vi "LSMcontroller_v63_3Dfocus.vi"() -> ()   [LabVIEW 2015] (continued)
                    n3072 = property on="save\ndata" class="Bool (strict)"("DisabledEnum"=T7."Enabled" ("Disabled")) -> ()  [unwired: 2 in, 2 out]
                    n3073 = property on="save\ndata" class="Bool (strict)"("Value"=TRUE ("save\ndata")) -> ()  [unwired: 2 in, 2 out]
                    n3074 = property on="# of frames" class="DigNum (strict)"("DisabledEnum"=T7."Enabled" ("Disabled")) -> ()  [unwired: 2 in, 2 out]
                  }
                }
              }
              frame #1 {
                n3075 = local read "finite samples"() -> (w6248:bool)
                n3076 = local read "continuous"() -> (w6247:bool)
                n3077 = local read "wavdet"() -> (w6246:bool)
                n3078 = call "2pparameters.vi"("command"="get") -> ("params out"=w6242:T10)  [unwired: 1 in]
                n3079 = Bundle By Name(cluster=w6242, "finite"=w6248, "cont"=w6247, "wavdet"=w6246) -> (w6245:T10)
                n3080 = call "2pparameters.vi"("Params in"=w6245, "command"="set") -> ()  [unwired: 1 out]
              }
            }
          }
          event "continuous": Value Change {
            n3081 = event-data() -> ("NewVal"=w6249:bool)  [unwired: 1 in]
            n3082 = flat-sequence {
              tunnel: w6249 -> [w6250]
              frame #0 {
                n3083 = case shown="True" w6250 {
                  frame False {
                    n3084 = property on="finite samples" class="Bool (strict)"("Value"=TRUE ("finite samples for recording")) -> ()  [unwired: 2 in, 2 out]
                    n3085 = property on="save\ndata" class="Bool (strict)"("Value"=TRUE ("save\ndata")) -> ()  [unwired: 2 in, 2 out]
                    n3086 = property on="wavdet" class="Bool (strict)"("Value"=FALSE ("wavdet")) -> ()  [unwired: 2 in, 2 out]
                    n3087 = local write "Save tab"(enum32{"withsave", "withoutsave"}."withsave" ("Save tab")) -> ()
                    n3088 = property on="# of frames" class="DigNum (strict)"("DisabledEnum"=T7."Enabled" ("Disabled")) -> ()  [unwired: 2 in, 2 out]
                    n3089 = property on="save\ndata" class="Bool (strict)"("DisabledEnum"=T7."Enabled" ("Disabled")) -> ()  [unwired: 2 in, 2 out]
                  }
                  frame True {
                    w6257 = FALSE ("finite samples for recording")
                    n3090 = property on="finite samples" class="Bool (strict)"("Value"=w6257) -> ()  [unwired: 2 in, 2 out]
                    n3091 = property on="wavdet" class="Bool (strict)"("Value"=w6257) -> ()  [unwired: 2 in, 2 out]
                    n3092 = property on="save\ndata" class="Bool (strict)"("Value"=w6257) -> ()  [unwired: 2 in, 2 out]
                    n3093 = local write "Save tab"(enum32{"withsave", "withoutsave"}."withsave" ("Save tab")) -> ()
                    n3094 = property on="# of frames" class="DigNum (strict)"("DisabledEnum"=T7."Disabled and Grayed Out" ("Disabled")) -> ()  [unwired: 2 in, 2 out]
                    n3095 = property on="save\ndata" class="Bool (strict)"("DisabledEnum"=T7."Disabled and Grayed Out" ("Disabled")) -> ()  [unwired: 2 in, 2 out]
                  }
                }
              }
              frame #1 {
                n3096 = local read "finite samples"() -> (w6267:bool)
                n3097 = local read "continuous"() -> (w6266:bool)
                n3098 = local read "wavdet"() -> (w6265:bool)
                n3099 = call "2pparameters.vi"("command"="get") -> ("params out"=w6261:T10)  [unwired: 1 in]
                n3100 = Bundle By Name(cluster=w6261, "finite"=w6267, "cont"=w6266, "wavdet"=w6265) -> (w6264:T10)
                n3101 = call "2pparameters.vi"("Params in"=w6264, "command"="set") -> ()  [unwired: 1 out]
              }
            }
          }
          event "wavdet": Value Change {
            n3102 = event-data() -> ("NewVal"=w6268:bool)  [unwired: 1 in]
            n3103 = flat-sequence {
              tunnel: w6268 -> [w6269]
              frame #0 {
                n3104 = case shown="False" w6269 {
                  frame False {
                    n3105 = property on="finite samples" class="Bool (strict)"("Value"=TRUE ("finite samples for recording")) -> ()  [unwired: 2 in, 2 out]
                    n3106 = property on="continuous" class="Bool (strict)"("Value"=FALSE ("continuous")) -> ()  [unwired: 2 in, 2 out]
                    n3107 = local write "Save tab"(enum32{"withsave", "withoutsave"}."withsave" ("Save tab")) -> ()
                    n3108 = property on="save\ndata" class="Bool (strict)"("DisabledEnum"=T7."Enabled" ("Disabled")) -> ()  [unwired: 2 in, 2 out]
                    n3109 = property on="# of frames" class="DigNum (strict)"("DisabledEnum"=T7."Enabled" ("Disabled")) -> ()  [unwired: 2 in, 2 out]
                    n3110 = property on="save\ndata" class="Bool (strict)"("Value"=TRUE ("save\ndata")) -> ()  [unwired: 2 in, 2 out]
                  }
                  frame True {
                    w6278 = FALSE ("finite samples for recording")
                    n3111 = property on="finite samples" class="Bool (strict)"("Value"=w6278) -> ()  [unwired: 2 in, 2 out]
                    n3112 = property on="continuous" class="Bool (strict)"("Value"=w6278) -> ()  [unwired: 2 in, 2 out]
                    n3113 = property on="save\ndata" class="Bool (strict)"("DisabledEnum"=T7."Enabled" ("Disabled")) -> ()  [unwired: 2 in, 2 out]
                    n3114 = local write "Save tab"(enum32{"withsave", "withoutsave"}."withsave" ("Save tab")) -> ()
                    n3115 = property on="# of frames" class="DigNum (strict)"("DisabledEnum"=T7."Disabled" ("Disabled")) -> ()  [unwired: 2 in, 2 out]
                    n3116 = property on="save\ndata" class="Bool (strict)"("Value"=TRUE ("save\ndata")) -> ()  [unwired: 2 in, 2 out]
                  }
                }
              }
              frame #1 {
                n3117 = local read "finite samples"() -> (w6281:bool)
                n3118 = local read "continuous"() -> (w6282:bool)
                n3119 = local read "wavdet"() -> (w6283:bool)
                n3120 = call "2pparameters.vi"("command"="get") -> ("params out"=w6287:T10)  [unwired: 1 in]
                n3121 = Bundle By Name(cluster=w6287, "finite"=w6281, "cont"=w6282, "wavdet"=w6283) -> (w6284:T10)
                n3122 = call "2pparameters.vi"("Params in"=w6284, "command"="set") -> ()  [unwired: 1 out]
              }
            }
          }
          event "cursors": Value Change {
            n3123 = event-data() -> ()  [unwired: 1 in, 5 out]
            n3124 = case shown="True" "cursors" {
              frame False {
                n3125 = property on="img_CH1" class="IntGraph (strict)"("Active Cursor"=u32 0, "Cursor.Cursor Style"=u8 0 ("Cursor Style"), "Cursor.Cursor Point Style"=u8 0 ("Cursor Point Style")) -> ("Cursor.Cursor Position:Cursor X"=w6292:dbl, "Cursor.Cursor Position:Cursor Y"=w6293:dbl)  [unwired: 2 in, 2 out]
                n3126 = property on="img_CH2" class="IntGraph (strict)"("Active Cursor"=u32 0, "Cursor.Cursor Style"=u8 0 ("Cursor Style"), "Cursor.Cursor Point Style"=u8 0 ("Cursor Point Style")) -> ()  [unwired: 2 in, 2 out]
                n3127 = local write "cursor x [pixel]"(w6292) -> ()
                n3128 = local write "cursor y [pixel]"(w6293) -> ()
              }
              frame True {
                n3129 = stacked-sequence {
                  frame #0 {
                    n3130 = call "2pparameters.vi"("command"="get") -> ("params out"=w6308:T10)  [unwired: 1 in]
                    n3131 = Unbundle By Name(w6308) -> ("Xpixels Img"=w6309:i32, "Ypixels Img"=w6306:i32)
                    n3132 = To Double Precision Float(number=w6306) -> (double precision float=w6300:dbl)
                    n3133 = To Double Precision Float(number=w6309) -> (double precision float=w6305:dbl)
                    n3134 = Divide(x=w6300, y=2.0) -> (x/y=w6301:dbl)
                    n3135 = Divide(x=w6305, y=2.0) -> (x/y=w6303:dbl)
                    n3136 = Round To Nearest(number=w6301) -> (nearest integer value=w6299:dbl)
                    n3137 = Round To Nearest(number=w6303) -> (nearest integer value=w6302:dbl)
                    n3138 = property on="img_CH1" class="IntGraph (strict)"("Active Cursor"=u32 0, "Cursor.Cursor Style"=u8 8 ("Cursor Style"), "Cursor.Cursor Point Style"=u8 5 ("Cursor Point Style"), "Cursor.Cursor Position:Cursor X"=w6302, "Cursor.Cursor Position:Cursor Y"=w6299, "Cursor.Visible"=TRUE) -> ()  [unwired: 2 in, 2 out]
                  }
                  frame #1 {
                    n3139 = call "2pparameters.vi"("command"="get") -> ("params out"=w6328:T10)  [unwired: 1 in]
                    n3140 = call "2pparameters.vi"("command"="get") -> ("params out"=w6326:T10)  [unwired: 1 in]
                    n3141 = property on="img_CH1" class="IntGraph (strict)"("Active Cursor"=u32 0, "Cursor.Cursor Style"=u8 8 ("Cursor Style"), "Cursor.Cursor Point Style"=u8 5 ("Cursor Point Style")) -> ("Cursor.Cursor Position:Cursor X"=w6321:dbl, "Cursor.Cursor Position:Cursor Y"=w6320:dbl, "Cursor.Cursor Index"=w6343:i32, "Cursor.Cursor Plot"=w6342:i32, "Cursor.Visible"=w6313:bool)  [unwired: 2 in, 2 out]
                    "cursor x [pixel]" <- w6321
                    "cursor y [pixel]" <- w6320
                    n3142 = Unbundle By Name(w6328) -> ("Vy-max Img"=w6330:dbl, "Vy-min Img"=w6317:dbl, "Ypixels Img"=w6332:i32)
                    n3143 = Unbundle By Name(w6326) -> ("VX-max Img"=w6327:dbl, "Vx-min Img"=w6315:dbl, "Xpixels Img"=w6331:i32)
                    n3144 = Subtract(x=w6330, y=w6317) -> (x-y=w6335:dbl)
                    n3145 = Subtract(x=w6327, y=w6315) -> (x-y=w6333:dbl)
                    n3146 = local read "img_CH2"() -> (w6339:sgl[][])
                    n3147 = To Double Precision Float(number=w6331) -> (double precision float=w6334:dbl)
                    n3148 = local read "img_CH1"() -> (w6340:sgl[][])
                    n3149 = To Double Precision Float(number=w6332) -> (double precision float=w6336:dbl)
                    n3150 = Index Array(array=w6340, index (row)=w6343, index (col)=w6342) -> (element=→"value CH 1":sgl)
                    n3151 = Index Array(array=w6339, index (row)=w6343, index (col)=w6342) -> (element=→"value CH 2":sgl)
                    n3152 = Divide(x=w6333, y=w6334) -> (x/y=w6337:dbl)
                    n3153 = Divide(x=w6335, y=w6336) -> (x/y=w6338:dbl)
                    n3154 = Multiply(x=w6321, y=w6337) -> (x*y=w6316:dbl)
                    n3155 = Multiply(x=w6320, y=w6338) -> (x*y=w6319:dbl)
                    n3156 = property on="img_CH2" class="IntGraph (strict)"("Active Cursor"=u32 0, "Cursor.Cursor Style"=u8 8 ("Cursor Style"), "Cursor.Cursor Point Style"=u8 5 ("Cursor Point Style"), "Cursor.Cursor Position:Cursor X"=w6321, "Cursor.Cursor Position:Cursor Y"=w6320, "Cursor.Visible"=w6313) -> ()  [unwired: 2 in, 2 out]
                    n3157 = Add(x=w6316, y=w6315) -> (x+y=w6314:dbl)
                    n3158 = Add(x=w6319, y=w6317) -> (x+y=w6318:dbl)
                    n3159 = local write "Vx-ref"(w6314) -> ()
                    n3160 = local write "Vy-ref"(w6318) -> ()
                  }
                }
              }
            }
          }
          event "img_CH1": Cursor Move {
            n3161 = event-data() -> ("CursIdx"=w6348:i32)  [unwired: 1 in]
            n3162 = Equal To 0?(x=w6348) -> (x = 0?=w6349:bool)
            n3163 = case shown="True" w6349 {
              frame False {
              }
              frame True {
                n3164 = call "2pparameters.vi"("command"="get") -> ("params out"=w6369:T10)  [unwired: 1 in]
                n3165 = call "2pparameters.vi"("command"="get") -> ("params out"=w6371:T10)  [unwired: 1 in]
                n3166 = property on="img_CH1" class="IntGraph (strict)"("Active Cursor"=u32 0, "Cursor.Cursor Style"=u8 8 ("Cursor Style"), "Cursor.Cursor Point Style"=u8 5 ("Cursor Point Style")) -> ("Cursor.Cursor Position:Cursor X"=w6358:dbl, "Cursor.Cursor Position:Cursor Y"=w6357:dbl, "Cursor.Cursor Plot"=w6377:i32, "Cursor.Cursor Index"=w6376:i32, "Cursor.Visible"=w6350:bool)  [unwired: 2 in, 2 out]
                n3167 = Unbundle By Name(w6369) -> ("Vy-max Img"=w6367:dbl, "Vy-min Img"=w6356:dbl, "Ypixels Img"=w6365:i32)
                n3168 = Unbundle By Name(w6371) -> ("VX-max Img"=w6370:dbl, "Vx-min Img"=w6351:dbl, "Xpixels Img"=w6366:i32)
                n3169 = Subtract(x=w6367, y=w6356) -> (x-y=w6362:dbl)
                n3170 = Subtract(x=w6370, y=w6351) -> (x-y=w6364:dbl)
                n3171 = local write "cursor x [pixel]"(w6358) -> ()
                n3172 = local write "cursor y [pixel]"(w6357) -> ()
                n3173 = To Double Precision Float(number=w6366) -> (double precision float=w6363:dbl)
                n3174 = To Double Precision Float(number=w6365) -> (double precision float=w6361:dbl)
                n3175 = local read "img_CH2"() -> (w6378:sgl[][])
                n3176 = local read "img_CH1"() -> (w6381:sgl[][])
                n3177 = Index Array(array=w6378, index (row)=w6377, index (col)=w6376) -> (element=w6379:sgl)
                n3178 = Index Array(array=w6381, index (row)=w6377, index (col)=w6376) -> (element=w6380:sgl)
                n3179 = Divide(x=w6364, y=w6363) -> (x/y=w6360:dbl)
                n3180 = Divide(x=w6362, y=w6361) -> (x/y=w6359:dbl)
                n3181 = local write "value CH 2"(w6379) -> ()
                n3182 = Multiply(x=w6358, y=w6360) -> (x*y=w6353:dbl)
                n3183 = local write "value CH 1"(w6380) -> ()
                n3184 = Multiply(x=w6357, y=w6359) -> (x*y=w6355:dbl)
                n3185 = Add(x=w6353, y=w6351) -> (x+y=w6352:dbl)
                n3186 = local write "Vx-ref"(w6352) -> ()
                n3187 = Add(x=w6355, y=w6356) -> (x+y=w6354:dbl)
                n3188 = property on="img_CH2" class="IntGraph (strict)"("Active Cursor"=u32 0, "Cursor.Cursor Style"=u8 8 ("Cursor Style"), "Cursor.Cursor Point Style"=u8 5 ("Cursor Point Style"), "Cursor.Cursor Position:Cursor X"=w6358, "Cursor.Cursor Position:Cursor Y"=w6357, "Cursor.Visible"=w6350) -> ()  [unwired: 2 in, 2 out]
                n3189 = local write "Vy-ref"(w6354) -> ()
              }
            }
          }
          event "img_CH2": Cursor Move {
            n3190 = event-data() -> ("CursIdx"=w6385:i32)  [unwired: 1 in]
            n3191 = Equal To 0?(x=w6385) -> (x = 0?=w6386:bool)
            n3192 = case shown="True" w6386 {
              frame False {
              }
              frame True {
                n3193 = property on="img_CH2" class="IntGraph (strict)"("Active Cursor"=u32 0, "Cursor.Cursor Style"=u8 8 ("Cursor Style"), "Cursor.Cursor Point Style"=u8 5 ("Cursor Point Style")) -> ("Cursor.Cursor Position:Cursor X"=w6394:dbl, "Cursor.Cursor Position:Cursor Y"=w6395:dbl, "Cursor.Cursor Plot"=w6414:i32, "Cursor.Cursor Index"=w6413:i32, "Cursor.Visible"=w6387:bool)  [unwired: 2 in, 2 out]
                n3194 = call "2pparameters.vi"("command"="get") -> ("params out"=w6406:T10)  [unwired: 1 in]
                n3195 = call "2pparameters.vi"("command"="get") -> ("params out"=w6408:T10)  [unwired: 1 in]
                n3196 = local read "img_CH1"() -> (w6418:sgl[][])
                n3197 = local read "img_CH2"() -> (w6415:sgl[][])
                n3198 = local write "cursor x [pixel]"(w6394) -> ()
                n3199 = local write "cursor y [pixel]"(w6395) -> ()
                n3200 = Unbundle By Name(w6406) -> ("Vy-max Img"=w6404:dbl, "Vy-min Img"=w6389:dbl, "Ypixels Img"=w6402:i32)
                n3201 = Unbundle By Name(w6408) -> ("VX-max Img"=w6407:dbl, "Vx-min Img"=w6392:dbl, "Xpixels Img"=w6403:i32)
                n3202 = Index Array(array=w6418, index (row)=w6414, index (col)=w6413) -> (element=w6417:sgl)
                n3203 = Index Array(array=w6415, index (row)=w6414, index (col)=w6413) -> (element=w6416:sgl)
                n3204 = local write "value CH 2"(w6416) -> ()
                n3205 = local write "value CH 1"(w6417) -> ()
                n3206 = Subtract(x=w6404, y=w6389) -> (x-y=w6399:dbl)
                n3207 = Subtract(x=w6407, y=w6392) -> (x-y=w6401:dbl)
                n3208 = To Double Precision Float(number=w6403) -> (double precision float=w6400:dbl)
                n3209 = To Double Precision Float(number=w6402) -> (double precision float=w6398:dbl)
                n3210 = Divide(x=w6401, y=w6400) -> (x/y=w6397:dbl)
                n3211 = Divide(x=w6399, y=w6398) -> (x/y=w6396:dbl)
                n3212 = Multiply(x=w6394, y=w6397) -> (x*y=w6393:dbl)
                n3213 = Multiply(x=w6395, y=w6396) -> (x*y=w6390:dbl)
                n3214 = property on="img_CH1" class="IntGraph (strict)"("Active Cursor"=u32 0, "Cursor.Cursor Style"=u8 8 ("Cursor Style"), "Cursor.Cursor Point Style"=u8 5 ("Cursor Point Style"), "Cursor.Cursor Position:Cursor X"=w6394, "Cursor.Cursor Position:Cursor Y"=w6395, "Cursor.Visible"=w6387) -> ()  [unwired: 2 in, 2 out]
                n3215 = Add(x=w6393, y=w6392) -> (x+y=→"Vx-ref":dbl)
                n3216 = Add(x=w6390, y=w6389) -> (x+y=→"Vy-ref":dbl)
              }
            }
          }
          event "Focus": Value Change {
            n3217 = event-data() -> ()  [unwired: 1 in, 6 out]
            n3218 = flat-sequence {
              frame #0 {
                n3219 = local read "Focus"() -> (w6422:bool)
                n3220 = case shown="True" w6422 {
                  frame False {
                  }
                  frame True {
                    n3221 = local read "Vx-ref"() -> (w6426:dbl)
                    n3222 = local read "Vy-ref"() -> (w6425:dbl)
                    n3223 = local read "zV"() -> (w6423:dbl)
                    n3224 = call "focusvi.vi"("zc"=w6423, "yc"=w6425, "xc"=w6426) -> ("finalz"=→"zV":dbl)
                  }
                }
              }
              frame #1 {
                n3225 = local write "Focus"(FALSE ("Focus")) -> ()
              }
            }
          }
          event "auto shutter": Value Change {
            n3226 = event-data() -> ()  [unwired: 1 in, 6 out]
            n3227 = call "2pparameters.vi"("command"="get") -> ("params out"=w6430:T10)  [unwired: 1 in]
            n3228 = in-place {
              n3229 = in-place-cluster #46(w6430) -> ()  [unwired: 1 out]
              n3230 = local read "auto shutter"() -> (w6432:bool)
              n3231 = in-place-cluster #46("autoshutter"=w6432) -> (w6428:T10)
            }
            n3232 = call "2pparameters.vi"("Params in"=w6428, "command"="set") -> ()  [unwired: 1 out]
          }
          event "auto OD": Value Change {
            n3233 = event-data() -> ()  [unwired: 1 in, 6 out]
            n3234 = call "2pparameters.vi"("command"="get") -> ("params out"=w6435:T10)  [unwired: 1 in]
            n3235 = in-place {
              n3236 = in-place-cluster #47(w6435) -> ()  [unwired: 1 out]
              n3237 = local read "auto OD"() -> (w6437:bool)
              n3238 = in-place-cluster #47("auto OD"=w6437) -> (w6433:T10)
            }
            n3239 = call "2pparameters.vi"("Params in"=w6433, "command"="set") -> ()  [unwired: 1 out]
          }
          event "ODfilt": Value Change {
            n3240 = event-data() -> ("OldVal"=w6438:u16)  [unwired: 1 in, 5 out]
            n3241 = local read "ODfilt"() -> (w6439:u16)
            n3242 = call "2pparameters.vi"("command"="get") -> ("params out"=w6442:T10)  [unwired: 1 in]
            n3243 = call "filterwheelcontrol_nothorlabslib.vi"("Current OD filt"=w6438, "New ODfilt"=w6439) -> ()  [unwired: 1 in]
            n3244 = in-place {
              in-place-border: w6439 -> [w6444]
              n3245 = in-place-cluster #48(w6442) -> ()  [unwired: 1 out]
              n3246 = in-place-cluster #48("ODfilt"=w6444) -> (w6440:T10)
            }
            n3247 = call "2pparameters.vi"("Params in"=w6440, "command"="set") -> ()  [unwired: 1 out]
          }
          event "Exit": Value Change {
            n3248 = event-data() -> ()  [unwired: 1 in, 5 out]
          }
        }
        n3249 = Wait (ms)(milliseconds to wait=u32 50) -> ()  [unwired: 1 out]
      }
      n3250 = while {
        stop <- w69 stop-if-true
        # "Waveform generation"
        n3251 = event shown="[2] \"AO channels\": Value Change" {
          selector: _ -> [_ _ _ _ _ _ _ _ _ _ _ _ _ _ _ _ _]
          dyn-events: _ -> [_ _ _ _ _ _ _ _ _ _ _ _ _ _ _ _ _]
          timeout: _ -> [_ _ _ _ _ _ _ _ _ _ _ _ _ _ _ _ _]
          tunnel: [_ _ _ _ _ _ _ _ _ _ _ _ _ _ _ _ w2042] -> w69
          event Timeout {
            n3252 = event-data() -> ()  [unwired: 1 in, 3 out]
          }
          event "Add AO wave": Value Change {
            n3253 = event-data() -> ("NewVal"=w70:bool)  [unwired: 1 in, 5 out]
            n3254 = case shown="True" w70 {
              frame False {
              }
              frame True {
                n3255 = stacked-sequence {
                  frame #0 {
                    n3256 = local read "Measurement"() -> (w71:T4)
                    n3257 = case shown="\"Lifetime (contour)\"" w71 {
                      frame "X-Y-t movie", Default {
                        n3258 = local read "avpp"() -> (w92:i32)
                        n3259 = local read "Angle ref"() -> (w91:dbl)
                        n3260 = local read "ROI Type"() -> (w90:u16)
                        n3261 = local read "xpixels ref"() -> (w87:i32)
                        n3262 = local read "Vx-min ref"() -> (w86:dbl)
                        n3263 = local read "Vx-max ref"() -> (w85:dbl)
                        n3264 = local read "ypixels ref"() -> (w83:i32)
                        n3265 = local read "Vy-min ref"() -> (w84:dbl)
                        n3266 = local read "Vy-max ref"() -> (w80:dbl)
                        n3267 = local read "Sampling rate"() -> (w74:dbl)
                        n3268 = local read "finite samples"() -> (w75:bool)
                        n3269 = local read "continuous"() -> (w78:bool)
                        n3270 = local read "wavdet"() -> (w79:bool)
                        n3271 = local read "# of frames"() -> (w77:i32)
                        n3272 = local read "maxbufferAI"() -> (w76:i32)
                        n3273 = local read "Override AI buffer"() -> (w72:bool)
                        n3274 = call "2pparameters.vi"("command"="get") -> ("params out"=w89:T10)  [unwired: 1 in]
                        n3275 = Bundle By Name(cluster=w89, "type"="X-Y-t movie", "avpp"=w92, "Angle Img"=w91, "Xpixels Img"=w87, "Vx-min Img"=w86, "VX-max Img"=w85, "Ypixels Img"=w83, "Vy-min Img"=w84, "Vy-max Img"=w80, "srate"=w74, "srate Img"=w74, "finite"=w75, "cont"=w78, "wavdet"=w79, "measpoints"=w77, "maxbufferAI"=w76, "Drawing Mode"=w90, "Vz-reset"=0.0, "AIoverride"=w72) -> (w81:T10)
                        n3276 = call "2pparameters.vi"("Params in"=w81, "command"="set") -> ()  [unwired: 1 out]
                      }
                      frame "X-Y-Z stack" {
                        n3277 = call "2pparameters.vi"("command"="get") -> ("params out"=w96:T10)  [unwired: 1 in]
                        n3278 = Bundle By Name(cluster=w96, "type"="X-Y-Z stack") -> (w94:T10)
                        n3279 = call "2pparameters.vi"("Params in"=w94, "command"="set") -> ()  [unwired: 1 out]
                      }
                      frame "Lifetime (scan)" {
                        n3280 = call "2pparameters.vi"("command"="get") -> ("params out"=w101:T10)  [unwired: 1 in]
                        n3281 = Bundle By Name(cluster=w101, "type"="Lifetime (scan)") -> (w99:T10)
                        n3282 = call "2pparameters.vi"("Params in"=w99, "command"="set") -> ()  [unwired: 1 out]
                      }
                      frame "Lifetime (contour)" {
                        n3283 = local read "Vy-min draw"() -> (w111:dbl)
                        n3284 = local read "Vy-max draw"() -> (w110:dbl)
                        n3285 = local read "Vx-min draw"() -> (w113:dbl)
                        n3286 = local read "Vx-max draw"() -> (w112:dbl)
                        n3287 = local read "xpixels ref"() -> (w109:i32)
                        n3288 = local read "ypixels ref"() -> (w108:i32)
                        n3289 = local read "ROI Type"() -> (w107:u16)
                        n3290 = local read "srateAODOtt"() -> (w118:dbl)
                        n3291 = local read "# of frames"() -> (w123:i32)
                        n3292 = local read "refreshtime"() -> (w115:dbl)
                        n3293 = local read "Pel"() -> (w106:dbl)
                        n3294 = local read "bin"() -> (w121:dbl)
                        n3295 = local read "Override AI buffer"() -> (w104:bool)
                        n3296 = local read "finite samples"() -> (w130:bool)
                        n3297 = local read "srateAODOtt"() -> (w117:dbl)
                        n3298 = local read "srateAODOtt"() -> (w124:dbl)
                        n3299 = local read "continuous"() -> (w129:bool)
                        n3300 = local read "Angle ref"() -> (w114:dbl)
                        n3301 = local read "wavdet"() -> (w131:bool)
                        n3302 = local read "Vx-ref"() -> (w126:dbl)
                        n3303 = local read "Vy-ref"() -> (w128:dbl)
                        n3304 = local read "avpp"() -> (w127:i32)
                        n3305 = call "tt_timeandsamples.vi"("bin"=w121, "refreshtime"=w115, "srateAODOtt"=w118, "tot#ofsamples"=w123) -> ("refreshrate"=w119:dbl, "refreshbuffer"=w120:i32, "timetracecycles"=w125:i32)  [unwired: 5 in]
                        n3306 = local read "bin"() -> (w122:dbl)
                        n3307 = call "2pparameters.vi"("command"="get") -> ("params out"=w134:T10)  [unwired: 1 in]
                        n3308 = Bundle By Name(cluster=w134, "Drawing Mode"=w107, "measpoints"=w123, "tt_cycles"=w125, "refreshbuffer"=w120, "refreshrate"=w119, "Vx-ref"=w126, "Vy-ref"=w128, "srate"=w117, "finite"=w130, "cont"=w129, "wavdet"=w131, "avpp"=w127, "srateAODO"=w124, "bufferAI"=w120, "bin"=w122, "Angle Img"=w114, "Vxminref"=w113, "Vxmaxref"=w112, "Vyminref"=w111, "Vymaxref"=w110, "Xpixels Img"=w109, "Ypixels Img"=w108, "Pel"=w106, "Vz-reset"=0.0, "AIoverride"=w104, "type"="Lifetime (contour)") -> (w132:T10)
                        n3309 = Reciprocal(x=w119) -> (1/x=w116:dbl)
                        n3310 = local write "refreshtime"(w116) -> ()
                        n3311 = call "2pparameters.vi"("Params in"=w132, "command"="set") -> ()  [unwired: 1 out]
                      }
                      frame "X-Y-Z-t movie" {
                      }
                      frame "linescan" {
                      }
                      frame "Timetrace" {
                        n3312 = local read "Vy-min draw"() -> (w144:dbl)
                        n3313 = local read "Vy-max draw"() -> (w143:dbl)
                        n3314 = local read "Vx-min draw"() -> (w146:dbl)
                        n3315 = local read "Vx-max draw"() -> (w145:dbl)
                        n3316 = local read "xpixels ref"() -> (w142:i32)
                        n3317 = local read "ypixels ref"() -> (w141:i32)
                        n3318 = local read "ROI Type"() -> (w140:u16)
                        n3319 = local read "srateAODOtt"() -> (w151:dbl)
                        n3320 = local read "# of frames"() -> (w156:i32)
                        n3321 = local read "refreshtime"() -> (w148:dbl)
                        n3322 = local read "Pel"() -> (w139:dbl)
                        n3323 = local read "bin"() -> (w154:dbl)
                        n3324 = local read "Override AI buffer"() -> (w137:bool)
                        n3325 = local read "finite samples"() -> (w163:bool)
                        n3326 = local read "srateAODOtt"() -> (w150:dbl)
                        n3327 = local read "srateAODOtt"() -> (w157:dbl)
                        n3328 = local read "continuous"() -> (w162:bool)
                        n3329 = local read "Angle ref"() -> (w147:dbl)
                        n3330 = local read "wavdet"() -> (w164:bool)
                        n3331 = local read "Vx-ref"() -> (w159:dbl)
                        n3332 = local read "Vy-ref"() -> (w161:dbl)
                        n3333 = local read "avpp"() -> (w160:i32)
                        n3334 = call "tt_timeandsamples.vi"("bin"=w154, "refreshtime"=w148, "srateAODOtt"=w151, "tot#ofsamples"=w156) -> ("refreshrate"=w152:dbl, "refreshbuffer"=w153:i32, "timetracecycles"=w158:i32)  [unwired: 5 in]
                        n3335 = local read "bin"() -> (w155:dbl)
                        n3336 = call "2pparameters.vi"("command"="get") -> ("params out"=w167:T10)  [unwired: 1 in]
                        n3337 = Bundle By Name(cluster=w167, "Drawing Mode"=w140, "measpoints"=w156, "tt_cycles"=w158, "refreshbuffer"=w153, "refreshrate"=w152, "Vx-ref"=w159, "Vy-ref"=w161, "srate"=w150, "finite"=w163, "cont"=w162, "wavdet"=w164, "avpp"=w160, "srateAODO"=w157, "bufferAI"=w153, "bin"=w155, "Angle Img"=w147, "Vxminref"=w146, "Vxmaxref"=w145, "Vyminref"=w144, "Vymaxref"=w143, "Xpixels Img"=w142, "Ypixels Img"=w141, "Pel"=w139, "Vz-reset"=0.0, "AIoverride"=w137, "type"="Timetrace") -> (w165:T10)
                        n3338 = Reciprocal(x=w152) -> (1/x=w149:dbl)
                        n3339 = local write "refreshtime"(w149) -> ()
                        n3340 = call "2pparameters.vi"("Params in"=w165, "command"="set") -> ()  [unwired: 1 out]
                      }
                      frame "Lifetime (point)" {
                      }
                    }
                  }
                  frame #1 {
                    w170 = FALSE ("wavdet")
                    n3341 = call "2pparameters.vi"("command"="get") -> ("params out"=w174:T10)  [unwired: 1 in]
                    n3342 = Bundle By Name(cluster=w174, "finite"=w170, "cont"=w170, "wavdet"=TRUE) -> (w171:T10)
                    n3343 = call "2pparameters.vi"("Params in"=w171, "command"="set") -> ()  [unwired: 1 out]
                  }
                  frame #2 {
                    # "change active waveform numbers array"
                    n3344 = local read "AO channels"() -> (w181:u32)
                    n3345 = call "2pparameters.vi"("command"="get") -> ("params out"=w179:T10)  [unwired: 1 in]
                    n3346 = in-place {
                      in-place-border: w181 -> [w185]
                      in-place-border: [w182] -> w176
                      n3347 = in-place-cluster #49(w179) -> ("aAO"=w184:u32[])
                      n3348 = call "add channel to active arrayv2.vi"("line array in"=w184, "line to add"=w185) -> ("line array out"=w183:u32[], "addition"=w182:bool)  [unwired: 1 out]
                      n3349 = in-place-cluster #49("aAO"=w183) -> (w177:T10)
                    }
                    n3350 = local write "addAO"(w176) -> ()
                    n3351 = call "2pparameters.vi"("Params in"=w177, "command"="set") -> ()  [unwired: 1 out]
                  }
                  frame #3 {
                    # "update GUI"
                    n3352 = local read "addAO"() -> (w186:bool)
                    n3353 = case shown="True" w186 {
                      frame False {
                      }
                      frame True {
                        n3354 = call "Used AO lines.vi"() -> ("used AO names"=w190:string[], "used AO lines"=w192:tag[])  [unwired: 2 in]
                        n3355 = control-ref of="Analog Lines Plot"() -> (w191:refnum<vi>)
                        n3356 = control-ref of="Digital Lines Plot"() -> (w189:refnum<vi>)
                        n3357 = call "Used DO lines.vi"() -> ("used DO names"=w188:string[], "used DO lines"=w187:tag[])  [unwired: 2 in]
                        n3358 = local write "Analog Used Lines"(w192) -> ()
                        n3359 = local write "Analog Used Names"(w190) -> ()
                        n3360 = local write "Digital Used Lines"(w187) -> ()
                        n3361 = local write "Digital Used Names"(w188) -> ()
                        n3362 = call "prepDOWaveplot.vi"("DigitalGraph in"=w189, "used DO names"=w188) -> ()  [unwired: 1 in]
                        n3363 = call "prepAOWaveplot.vi"("WaveformGraph in"=w191, "Analog Used Names"=w190) -> ()  [unwired: 1 in]
                      }
                    }
                  }
                  frame #4 {
                    n3364 = local read "addAO"() -> (w193:bool)
                    n3365 = case shown="True" w193 {
                      frame False {
                      }
                      frame True {
                        # "add parameters\nto parameter array"
                        n3366 = local read "Build analog waveform tabs"() -> (w194:enum32{"Square", "Triangle", "Matlab"})
                        n3367 = case shown="\"Square\", Default" w194 {
                          frame "Square", Default {
                            w207 = 0.0 ("Offset (V)")
                            n3368 = local read "Meastab"() -> (w196:enum32{"X-Y Image", "Linescan", "Timetrace"})
                            n3369 = call "waveformparamsv2.vi"("command"="get") -> ("Params out"=w205:T14)  [unwired: 4 in, 2 out]
                            n3370 = Unbundle By Name(w205) -> ("AO parameters"=w202:T15)
                            n3371 = case shown="\"Timetrace\"" w196 {
                              tunnel: [w218 w219] -> w195
                              frame "X-Y Image", Default {
                                n3372 = local read "Sampling rate"() -> (w218:dbl)
                              }
                              frame "Timetrace" {
                                n3373 = local read "srateAODOtt"() -> (w219:dbl)
                              }
                            }
                            n3374 = local read "Start amplitude (V)"() -> (w215:dbl)
                            n3375 = local read "phase shift (ms)"() -> (w208:dbl)
                            n3376 = local read "Step size (V)"() -> (w213:dbl)
                            n3377 = local read "Baseline (V)"() -> (w214:dbl)
                            n3378 = local read "Period (ms)"() -> (w211:dbl)
                            n3379 = local read "padding value"() -> (w198:dbl)
                            n3380 = local read "Repeats"() -> (w217:dbl)
                            n3381 = local read "DC (%)"() -> (w212:dbl)
                            n3382 = local read "Cycles"() -> (w216:dbl)
                            n3383 = local read "Pulses"() -> (w209:dbl)
                            n3384 = Index Array(array=w202, index=0) -> (element=w203:T16)
                            n3385 = Bundle By Name(cluster=w203, "AOtab"=0.0 ("Repeats"), "Repeats"=w217, "Cycles"=w216, "Start amplitude (V)"=w215, "Baseline (V)"=w214, "Step size (V)"=w213, "DC (%)"=w212, "Sampling frequency (Hz)"=w195, "Period (ms)"=w211, "Offset (V)"=w207, "Amplitude (V)"=w207, "Frequency"=w207, "Tri Repeats"=w207, "phase shift (ms)"=w208, "Pulses"=w209, "Matlab wave file"=path "", "padding value"=w198) -> (w200:T16)
                            n3386 = Build Array(w200) -> (w199:T15)
                            n3387 = call "waveformparamsv2.vi"("command"="add AO", "add AO"=w199) -> ()  [unwired: 3 in, 3 out]
                          }
                          frame "Matlab" {
                            w225 = 0.0 ("Repeats")
                            n3388 = local read "Meastab"() -> (w221:enum32{"X-Y Image", "Linescan", "Timetrace"})
                            n3389 = call "waveformparamsv2.vi"("command"="get") -> ("Params out"=w232:T14)  [unwired: 4 in, 2 out]
                            n3390 = Unbundle By Name(w232) -> ("AO parameters"=w229:T15)
                            n3391 = case shown="\"Timetrace\"" w221 {
                              tunnel: [w235 w236] -> w220
                              frame "X-Y Image", Default {
                                n3392 = local read "Sampling rate"() -> (w235:dbl)
                              }
                              frame "Timetrace" {
                                n3393 = local read "srateAODOtt"() -> (w236:dbl)
                              }
                            }
                            n3394 = local read "Matlab waveform path"() -> (w222:path)
                            n3395 = local read "Matlab padding value"() -> (w224:dbl)
                            n3396 = Index Array(array=w229, index=0) -> (element=w230:T16)
                            n3397 = call "matlabwfexistsdialogue.vi"("Matlab waveform path"=w222) -> ("mtalab waveform path out"=w223:path)
                            n3398 = Bundle By Name(cluster=w230, "AOtab"=2.0 ("Repeats"), "Repeats"=w225, "Cycles"=w225, "Start amplitude (V)"=w225, "Baseline (V)"=w225, "Step size (V)"=w225, "DC (%)"=w225, "Sampling frequency (Hz)"=w220, "Period (ms)"=w225, "Offset (V)"=w225, "Amplitude (V)"=w225, "Frequency"=w225, "Tri Repeats"=w225, "phase shift (ms)"=w225, "Pulses"=w225, "Matlab wave file"=w223, "padding value"=w224) -> (w227:T16)
                            n3399 = Build Array(w227) -> (w226:T15)
                            n3400 = call "waveformparamsv2.vi"("command"="add AO", "add AO"=w226) -> ()  [unwired: 3 in, 3 out]
                          }
                          frame "Triangle" {
                            w242 = 0.0 ("Offset (V)")
                            n3401 = local read "Meastab"() -> (w238:enum32{"X-Y Image", "Linescan", "Timetrace"})
                            n3402 = call "waveformparamsv2.vi"("command"="get") -> ("Params out"=w254:T14)  [unwired: 4 in, 2 out]
                            n3403 = Unbundle By Name(w254) -> ("AO parameters"=w251:T15)
                            n3404 = case shown="\"Timetrace\"" w238 {
                              tunnel: [w256 w257] -> w237
                              frame "X-Y Image", Default {
                                n3405 = local read "Sampling rate"() -> (w256:dbl)
                              }
                              frame "Timetrace" {
                                n3406 = local read "srateAODOtt"() -> (w257:dbl)
                              }
                            }
                            n3407 = local read "Tri padding value"() -> (w240:dbl)
                            n3408 = local read "Amplitude (V)"() -> (w245:dbl)
                            n3409 = local read "Tri Phase (s)"() -> (w241:dbl)
                            n3410 = local read "Tri Repeats"() -> (w243:dbl)
                            n3411 = local read "Frequency"() -> (w244:dbl)
                            n3412 = local read "Offset (V)"() -> (w246:dbl)
                            n3413 = Index Array(array=w251, index=0) -> (element=w252:T16)
                            n3414 = Bundle By Name(cluster=w252, "AOtab"=1.0 ("Repeats"), "Repeats"=w242, "Cycles"=w242, "Start amplitude (V)"=w242, "Baseline (V)"=w242, "Step size (V)"=w242, "DC (%)"=w242, "Sampling frequency (Hz)"=w237, "Period (ms)"=w242, "Offset (V)"=w246, "Amplitude (V)"=w245, "Frequency"=w244, "Tri Repeats"=w243, "phase shift (ms)"=w242, "Pulses"=w242, "Matlab wave file"=path "", "Tri phase"=w241, "padding value"=w240) -> (w249:T16)
                            n3415 = Build Array(w249) -> (w248:T15)
                            n3416 = call "waveformparamsv2.vi"("command"="add AO", "add AO"=w248) -> ()  [unwired: 3 in, 3 out]
                          }
                        }
                      }
                    }
                  }
                  frame #5 {
                    n3417 = local read "addAO"() -> (w258:bool)
                    n3418 = case shown="True" w258 {
                      frame False {
                      }
                      frame True {
                        # "add waveform to waveform array; correct waveform lengths and plot"
                        n3419 = local read "Meastab"() -> (w262:enum32{"X-Y Image", "Linescan", "Timetrace"})
                        n3420 = local read "Build analog waveform tabs"() -> (w272:enum32{"Square", "Triangle", "Matlab"})
                        n3421 = case shown="\"Timetrace\"" w262 {
                          tunnel: [w280 w281] -> w261
                          frame "X-Y Image", Default {
                            n3422 = local read "Sampling rate"() -> (w280:dbl)
                          }
                          frame "Timetrace" {
                            n3423 = local read "srateAODOtt"() -> (w281:dbl)
                          }
                        }
                        n3424 = call "waveformparamsv2.vi"("command"="get last AO") -> ("last AO"=w274:T16)  [unwired: 4 in, 2 out]
                        n3425 = case shown="\"Matlab\"" w272 {
                          tunnel: w274 -> [w284 w286 w288]
                          tunnel: [w283 w285 w287] -> w273
                          frame "Square", Default {
                            n3426 = call "generateRampedSquareWave_fromAOparameters.vi"("AO params"=w284) -> ("Waveform"=w283:waveform(dbl))  [unwired: 1 out]
                          }
                          frame "Triangle" {
                            n3427 = call "generateTriWave_fromAOparameters.vi"("AO params"=w286) -> ("Waveform"=w285:waveform(dbl))  [unwired: 1 out]
                          }
                          frame "Matlab" {
                            n3428 = call "matlabAOwffromparam.vi"("Cluster"=w288) -> ("Waveform"=w287:waveform(dbl))  [unwired: 1 out]
                          }
                        }
                        n3429 = property on="refwf" class="Ring (strict)"() -> ("RingText.Text"=w265:string)  [unwired: 2 in, 2 out]
                        n3430 = call "waveformsAObuffer.vi"("command"="get") -> ("AO wf out"=w278:waveform(dbl)[])  [unwired: 1 in]
                        n3431 = Build Array (concatenate)(w278, w273) -> (w275:waveform(dbl)[])
                        n3432 = call "waveformsDObuffer.vi"("command"="get") -> ("DO wf out"=w270:digitalwaveform[])  [unwired: 1 in]
                        n3433 = call "correctwaveformsizetemp.vi"("new sampling frequency (Hz)"=w261, "start"=FALSE, "reference waveforms to"=w265, "Analog waveforms in"=w275, "stop"=FALSE, "Digital waveforms in"=w270) -> ("analog wf out"=w268:waveform(dbl)[], "Digital wf out"=w266:digitalwaveform[], "measpoints"=w263:i32)
                        n3434 = local write "Analog Lines Plot"(w268) -> ()
                        n3435 = call "GetNumCamFramesv2.vi"("Digital Waveform Graph"=w266) -> ("Numeric"=w267:i32)  [unwired: 10 in]
                        n3436 = local write "Digital Lines Plot"(w266) -> ()
                        n3437 = call "waveformsAObuffer.vi"("AO wf in"=w268, "command"="set") -> ()  [unwired: 1 out]
                        n3438 = call "waveformsDObuffer.vi"("DO wf in"=w266, "command"="set") -> ()  [unwired: 1 out]
                        n3439 = local write "Total Camera Frames"(w267) -> ()
                        n3440 = local read "wavdet"() -> (w264:bool)
                        n3441 = case shown="True" w264 {
                          tunnel: w263 -> [_ w282]
                          frame False {
                          }
                          frame True {
                            n3442 = local write "# of frames"(w282) -> ()
                          }
                        }
                      }
                    }
                  }
                  frame #6 {
                    w289 = FALSE ("addAO")
                    # "set signaling boolean to false"
                    n3443 = local read "finite samples"() -> (w290:bool)
                    n3444 = local read "continuous"() -> (w291:bool)
                    n3445 = local read "wavdet"() -> (w292:bool)
                    n3446 = call "2pparameters.vi"("command"="get") -> ("params out"=w295:T10)  [unwired: 1 in]
                    n3447 = Bundle By Name(cluster=w295, "finite"=w290, "cont"=w291, "wavdet"=w292) -> (w293:T10)
                    n3448 = local write "addAO"(w289) -> ()
                    n3449 = property on="Add AO wave" class="Bool (strict)"("Val(Sgnl)"=w289) -> ()  [unwired: 2 in, 2 out]
                    n3450 = call "2pparameters.vi"("Params in"=w293, "command"="set") -> ()  [unwired: 1 out]
                  }
                }
              }
            }
          }
          event "AO channels": Value Change {
            n3451 = event-data() -> ()  [unwired: 1 in, 6 out]
            n3452 = local read "AO channels"() -> (w297:u32)
            n3453 = call "2pparameters.vi"("command"="get") -> ("params out"=w299:T10)  [unwired: 1 in]
            n3454 = Unbundle By Name(w299) -> ("aAO"=w298:u32[])
            n3455 = Search 1D Array(1D array=w298, element=w297) -> (index of element=w301:i32)  [unwired: 1 in]
            n3456 = Equal?(x=w301, y=-1.0) -> (x = y?=w302:bool)
            n3457 = case shown="False" w302 {
              tunnel: w301 -> [w304 _]
              frame False {
                n3458 = call "waveformparamsv2.vi"("command"="get") -> ("Params out"=w311:T14)  [unwired: 4 in, 2 out]
                n3459 = Unbundle By Name(w311) -> ("AO parameters"=w310:T15)
                n3460 = Index Array(array=w310, index=w304) -> (element=w327:T16)
                n3461 = Unbundle By Name(w327) -> ("AOtab"=w308:dbl, "Repeats"=w326:dbl, "Cycles"=w325:dbl, "Start amplitude (V)"=w324:dbl, "Baseline (V)"=w323:dbl, "Step size (V)"=w322:dbl, "DC (%)"=w321:dbl, "Sampling frequency (Hz)"=w320:dbl, "Period (ms)"=w319:dbl, "Offset (V)"=w318:dbl, "Amplitude (V)"=w317:dbl, "Frequency"=w316:dbl, "Tri Repeats"=w315:dbl, "phase shift (ms)"=w314:dbl, "Pulses"=w313:dbl, "Tri phase"=w309:dbl, "padding value"=w305:dbl, "Matlab wave file"=w306:path)
                n3462 = To Unsigned Long Integer(number=w308) -> (unsigned 32bit integer=w307:u32)
                n3463 = local write "Build analog waveform tabs"(w307) -> ()
                n3464 = local write "Matlab waveform path"(w306) -> ()
                n3465 = local write "phase shift (ms)"(w314) -> ()
                n3466 = local write "Repeats"(w326) -> ()
                n3467 = local write "Cycles"(w325) -> ()
                n3468 = local write "Amplitude (V)"(w317) -> ()
                n3469 = local write "Matlab padding value"(w305) -> ()
                n3470 = local write "Tri padding value"(w305) -> ()
                n3471 = local write "Start amplitude (V)"(w324) -> ()
                n3472 = local write "Tri Phase (s)"(w309) -> ()
                n3473 = local write "Period (ms)"(w319) -> ()
                n3474 = local write "Tri Repeats"(w315) -> ()
                n3475 = local write "Offset (V)"(w318) -> ()
                n3476 = local write "Frequency"(w316) -> ()
                n3477 = local write "Pulses"(w313) -> ()
                n3478 = local write "padding value"(w305) -> ()
                n3479 = local write "Sampling rate \ncurrent wf"(w320) -> ()
                n3480 = local write "Baseline (V)"(w323) -> ()
                n3481 = local write "Step size (V)"(w322) -> ()
                n3482 = local write "DC (%)"(w321) -> ()
              }
              frame True {
              }
            }
          }
          event "Rem AO wave": Value Change {
            n3483 = event-data() -> ("NewVal"=w328:bool)  [unwired: 1 in, 5 out]
            n3484 = case shown="True" w328 {
              frame False {
              }
              frame True {
                n3485 = stacked-sequence {
                  seq-local: [_ _ w434 _ _ _ _] -> [_ _ _ _ w454 w457 _]
                  frame #0 {
                    n3486 = local read "Measurement"() -> (w329:T4)
                    n3487 = case shown="\"X-Y-t movie\", Default" w329 {
                      frame "X-Y-t movie", Default {
                        n3488 = local read "avpp"() -> (w350:i32)
                        n3489 = local read "Angle ref"() -> (w349:dbl)
                        n3490 = local read "ROI Type"() -> (w348:u16)
                        n3491 = local read "xpixels ref"() -> (w345:i32)
                        n3492 = local read "Vx-min ref"() -> (w344:dbl)
                        n3493 = local read "Vx-max ref"() -> (w343:dbl)
                        n3494 = local read "ypixels ref"() -> (w341:i32)
                        n3495 = local read "Vy-min ref"() -> (w342:dbl)
                        n3496 = local read "Vy-max ref"() -> (w338:dbl)
                        n3497 = local read "Sampling rate"() -> (w332:dbl)
                        n3498 = local read "finite samples"() -> (w333:bool)
                        n3499 = local read "continuous"() -> (w336:bool)
                        n3500 = local read "wavdet"() -> (w337:bool)
                        n3501 = local read "# of frames"() -> (w335:i32)
                        n3502 = local read "maxbufferAI"() -> (w334:i32)
                        n3503 = local read "Override AI buffer"() -> (w330:bool)
                        n3504 = call "2pparameters.vi"("command"="get") -> ("params out"=w347:T10)  [unwired: 1 in]
                        n3505 = Bundle By Name(cluster=w347, "type"="X-Y-t movie", "avpp"=w350, "Angle Img"=w349, "Xpixels Img"=w345, "Vx-min Img"=w344, "VX-max Img"=w343, "Ypixels Img"=w341, "Vy-min Img"=w342, "Vy-max Img"=w338, "srate"=w332, "srate Img"=w332, "finite"=w333, "cont"=w336, "wavdet"=w337, "measpoints"=w335, "maxbufferAI"=w334, "Drawing Mode"=w348, "Vz-reset"=0.0, "AIoverride"=w330) -> (w339:T10)
                        n3506 = call "2pparameters.vi"("Params in"=w339, "command"="set") -> ()  [unwired: 1 out]
                      }
                      frame "X-Y-Z stack" {
                        n3507 = call "2pparameters.vi"("command"="get") -> ("params out"=w354:T10)  [unwired: 1 in]
                        n3508 = Bundle By Name(cluster=w354, "type"="X-Y-Z stack") -> (w352:T10)
                        n3509 = call "2pparameters.vi"("Params in"=w352, "command"="set") -> ()  [unwired: 1 out]
                      }
                      frame "Lifetime (scan)" {
                        n3510 = call "2pparameters.vi"("command"="get") -> ("params out"=w359:T10)  [unwired: 1 in]
                        n3511 = Bundle By Name(cluster=w359, "type"="Lifetime (scan)") -> (w357:T10)
                        n3512 = call "2pparameters.vi"("Params in"=w357, "command"="set") -> ()  [unwired: 1 out]
                      }
                      frame "Lifetime (contour)" {
                        n3513 = local read "Vy-min draw"() -> (w369:dbl)
                        n3514 = local read "Vy-max draw"() -> (w368:dbl)
                        n3515 = local read "Vx-min draw"() -> (w371:dbl)
                        n3516 = local read "Vx-max draw"() -> (w370:dbl)
                        n3517 = local read "xpixels ref"() -> (w367:i32)
                        n3518 = local read "ypixels ref"() -> (w366:i32)
                        n3519 = local read "ROI Type"() -> (w365:u16)
                        n3520 = local read "srateAODOtt"() -> (w376:dbl)
                        n3521 = local read "# of frames"() -> (w381:i32)
                        n3522 = local read "refreshtime"() -> (w373:dbl)
                        n3523 = local read "Pel"() -> (w364:dbl)
                        n3524 = local read "bin"() -> (w379:dbl)
                        n3525 = local read "Override AI buffer"() -> (w362:bool)
                        n3526 = local read "finite samples"() -> (w388:bool)
                        n3527 = local read "srateAODOtt"() -> (w375:dbl)
                        n3528 = local read "srateAODOtt"() -> (w382:dbl)
                        n3529 = local read "continuous"() -> (w387:bool)
                        n3530 = local read "Angle ref"() -> (w372:dbl)
                        n3531 = local read "wavdet"() -> (w389:bool)
                        n3532 = local read "Vx-ref"() -> (w384:dbl)
                        n3533 = local read "Vy-ref"() -> (w386:dbl)
                        n3534 = local read "avpp"() -> (w385:i32)
                        n3535 = call "tt_timeandsamples.vi"("bin"=w379, "refreshtime"=w373, "srateAODOtt"=w376, "tot#ofsamples"=w381) -> ("refreshrate"=w377:dbl, "refreshbuffer"=w378:i32, "timetracecycles"=w383:i32)  [unwired: 5 in]
                        n3536 = local read "bin"() -> (w380:dbl)
                        n3537 = call "2pparameters.vi"("command"="get") -> ("params out"=w392:T10)  [unwired: 1 in]
                        n3538 = Bundle By Name(cluster=w392, "Drawing Mode"=w365, "measpoints"=w381, "tt_cycles"=w383, "refreshbuffer"=w378, "refreshrate"=w377, "Vx-ref"=w384, "Vy-ref"=w386, "srate"=w375, "finite"=w388, "cont"=w387, "wavdet"=w389, "avpp"=w385, "srateAODO"=w382, "bufferAI"=w378, "bin"=w380, "Angle Img"=w372, "Vxminref"=w371, "Vxmaxref"=w370, "Vyminref"=w369, "Vymaxref"=w368, "Xpixels Img"=w367, "Ypixels Img"=w366, "Pel"=w364, "Vz-reset"=0.0, "AIoverride"=w362, "type"="Lifetime (contour)") -> (w390:T10)
                        n3539 = Reciprocal(x=w377) -> (1/x=w374:dbl)
                        n3540 = local write "refreshtime"(w374) -> ()
                        n3541 = call "2pparameters.vi"("Params in"=w390, "command"="set") -> ()  [unwired: 1 out]
                      }
                      frame "X-Y-Z-t movie" {
                      }
                      frame "linescan" {
                      }
                      frame "Timetrace" {
                        n3542 = local read "Vy-min draw"() -> (w402:dbl)
                        n3543 = local read "Vy-max draw"() -> (w401:dbl)
                        n3544 = local read "Vx-min draw"() -> (w404:dbl)
                        n3545 = local read "Vx-max draw"() -> (w403:dbl)
                        n3546 = local read "xpixels ref"() -> (w400:i32)
                        n3547 = local read "ypixels ref"() -> (w399:i32)
                        n3548 = local read "ROI Type"() -> (w398:u16)
                        n3549 = local read "srateAODOtt"() -> (w409:dbl)
                        n3550 = local read "# of frames"() -> (w414:i32)
                        n3551 = local read "refreshtime"() -> (w406:dbl)
                        n3552 = local read "Pel"() -> (w397:dbl)
                        n3553 = local read "bin"() -> (w412:dbl)
                        n3554 = local read "Override AI buffer"() -> (w395:bool)
                        n3555 = local read "finite samples"() -> (w421:bool)
                        n3556 = local read "srateAODOtt"() -> (w408:dbl)
                        n3557 = local read "srateAODOtt"() -> (w415:dbl)
                        n3558 = local read "continuous"() -> (w420:bool)
                        n3559 = local read "Angle ref"() -> (w405:dbl)
                        n3560 = local read "wavdet"() -> (w422:bool)
                        n3561 = local read "Vx-ref"() -> (w417:dbl)
                        n3562 = local read "Vy-ref"() -> (w419:dbl)
                        n3563 = local read "avpp"() -> (w418:i32)
                        n3564 = call "tt_timeandsamples.vi"("bin"=w412, "refreshtime"=w406, "srateAODOtt"=w409, "tot#ofsamples"=w414) -> ("refreshrate"=w410:dbl, "refreshbuffer"=w411:i32, "timetracecycles"=w416:i32)  [unwired: 5 in]
                        n3565 = local read "bin"() -> (w413:dbl)
                        n3566 = call "2pparameters.vi"("command"="get") -> ("params out"=w425:T10)  [unwired: 1 in]
                        n3567 = Bundle By Name(cluster=w425, "Drawing Mode"=w398, "measpoints"=w414, "tt_cycles"=w416, "refreshbuffer"=w411, "refreshrate"=w410, "Vx-ref"=w417, "Vy-ref"=w419, "srate"=w408, "finite"=w421, "cont"=w420, "wavdet"=w422, "avpp"=w418, "srateAODO"=w415, "bufferAI"=w411, "bin"=w413, "Angle Img"=w405, "Vxminref"=w404, "Vxmaxref"=w403, "Vyminref"=w402, "Vymaxref"=w401, "Xpixels Img"=w400, "Ypixels Img"=w399, "Pel"=w397, "Vz-reset"=0.0, "AIoverride"=w395, "type"="Timetrace") -> (w423:T10)
                        n3568 = Reciprocal(x=w410) -> (1/x=w407:dbl)
                        n3569 = local write "refreshtime"(w407) -> ()
                        n3570 = call "2pparameters.vi"("Params in"=w423, "command"="set") -> ()  [unwired: 1 out]
                      }
                      frame "Lifetime (point)" {
                      }
                    }
                  }
                  frame #1 {
                    w428 = FALSE ("wavdet")
                    n3571 = call "2pparameters.vi"("command"="get") -> ("params out"=w432:T10)  [unwired: 1 in]
                    n3572 = Bundle By Name(cluster=w432, "finite"=w428, "cont"=w428, "wavdet"=TRUE) -> (w429:T10)
                    n3573 = call "2pparameters.vi"("Params in"=w429, "command"="set") -> ()  [unwired: 1 out]
                  }
                  frame #2 {
                    # "remove channel from numbers array"
                    n3574 = local read "AO channels"() -> (w439:u32)
                    n3575 = call "2pparameters.vi"("command"="get") -> ("params out"=w437:T10)  [unwired: 1 in]
                    n3576 = in-place {
                      in-place-border: w439 -> [w445]
                      in-place-border: [w442] -> w440
                      in-place-border: [w441] -> w434
                      n3577 = in-place-cluster #50(w437) -> ("aAO"=w444:u32[])
                      n3578 = call "remove channel from active arrayv2.vi"("line array in"=w444, "line to remove"=w445) -> ("line array out"=w443:u32[], "removal"=w442:bool, "index"=w441:i32)
                      n3579 = in-place-cluster #50("aAO"=w443) -> (w435:T10)
                    }
                    n3580 = local write "remAO"(w440) -> ()
                    n3581 = call "2pparameters.vi"("Params in"=w435, "command"="set") -> ()  [unwired: 1 out]
                  }
                  frame #3 {
                    n3582 = local read "remAO"() -> (w446:bool)
                    n3583 = case shown="True" w446 {
                      frame False {
                      }
                      frame True {
                        n3584 = call "Used AO lines.vi"() -> ("used AO names"=w450:string[], "used AO lines"=w452:tag[])  [unwired: 2 in]
                        n3585 = control-ref of="Analog Lines Plot"() -> (w451:refnum<vi>)
                        n3586 = control-ref of="Digital Lines Plot"() -> (w449:refnum<vi>)
                        n3587 = call "Used DO lines.vi"() -> ("used DO names"=w448:string[], "used DO lines"=w447:tag[])  [unwired: 2 in]
                        n3588 = local write "Analog Used Lines"(w452) -> ()
                        n3589 = local write "Analog Used Names"(w450) -> ()
                        n3590 = local write "Digital Used Lines"(w447) -> ()
                        n3591 = local write "Digital Used Names"(w448) -> ()
                        n3592 = call "prepDOWaveplot.vi"("DigitalGraph in"=w449, "used DO names"=w448) -> ()  [unwired: 1 in]
                        n3593 = call "prepAOWaveplot.vi"("WaveformGraph in"=w451, "Analog Used Names"=w450) -> ()  [unwired: 1 in]
                      }
                    }
                  }
                  frame #4 {
                    n3594 = local read "remAO"() -> (w453:bool)
                    n3595 = case shown="True" w453 {
                      tunnel: w454 -> [_ w455]
                      frame False {
                      }
                      frame True {
                        n3596 = call "waveformparamsv2.vi"("command"="rem AO", "index"=w455) -> ()  [unwired: 3 in, 3 out]
                      }
                    }
                  }
                  frame #5 {
                    n3597 = local read "remAO"() -> (w458:bool)
                    n3598 = case shown="True" w458 {
                      tunnel: w457 -> [_ w477]
                      frame False {
                      }
                      frame True {
                        n3599 = local read "Meastab"() -> (w462:enum32{"X-Y Image", "Linescan", "Timetrace"})
                        n3600 = property on="refwf" class="Ring (strict)"() -> ("RingText.Text"=w465:string)  [unwired: 2 in, 2 out]
                        n3601 = case shown="\"Timetrace\"" w462 {
                          tunnel: [w478 w479] -> w461
                          frame "X-Y Image", Default {
                            n3602 = local read "Sampling rate"() -> (w478:dbl)
                          }
                          frame "Timetrace" {
                            n3603 = local read "srateAODOtt"() -> (w479:dbl)
                          }
                        }
                        n3604 = call "waveformsAObuffer.vi"("command"="get") -> ("AO wf out"=w474:waveform(dbl)[])  [unwired: 1 in]
                        n3605 = call "waveformsDObuffer.vi"("command"="get") -> ("DO wf out"=w471:digitalwaveform[])  [unwired: 1 in]
                        n3606 = Delete From Array(array=w474, length=1, index=w477) -> (array with subset deleted=w466:waveform(dbl)[])  [unwired: 1 out]
                        n3607 = call "correctwaveformsizetemp.vi"("new sampling frequency (Hz)"=w461, "start"=FALSE, "reference waveforms to"=w465, "Analog waveforms in"=w466, "stop"=FALSE, "Digital waveforms in"=w471) -> ("analog wf out"=w469:waveform(dbl)[], "Digital wf out"=w467:digitalwaveform[], "measpoints"=w463:i32)
                        n3608 = local write "Analog Lines Plot"(w469) -> ()
                        n3609 = call "GetNumCamFramesv2.vi"("Digital Waveform Graph"=w467) -> ("Numeric"=w468:i32)  [unwired: 10 in]
                        n3610 = local write "Digital Lines Plot"(w467) -> ()
                        n3611 = call "waveformsAObuffer.vi"("AO wf in"=w469, "command"="set") -> ()  [unwired: 1 out]
                        n3612 = call "waveformsDObuffer.vi"("DO wf in"=w467, "command"="set") -> ()  [unwired: 1 out]
                        n3613 = local read "wavdet"() -> (w464:bool)
                        n3614 = local write "Total Camera Frames"(w468) -> ()
                        n3615 = case shown="True" w464 {
                          tunnel: w463 -> [_ w480]
                          frame False {
                          }
                          frame True {
                            n3616 = local write "# of frames"(w480) -> ()
                          }
                        }
                      }
                    }
                  }
                  frame #6 {
                    w481 = FALSE ("remAO")
                    n3617 = local read "finite samples"() -> (w482:bool)
                    n3618 = local read "continuous"() -> (w483:bool)
                    n3619 = local read "wavdet"() -> (w484:bool)
                    n3620 = call "2pparameters.vi"("command"="get") -> ("params out"=w487:T10)  [unwired: 1 in]
                    n3621 = Bundle By Name(cluster=w487, "finite"=w482, "cont"=w483, "wavdet"=w484) -> (w485:T10)
                    n3622 = local write "remAO"(w481) -> ()
                    n3623 = property on="Rem AO wave" class="Bool (strict)"("Val(Sgnl)"=w481) -> ()  [unwired: 2 in, 2 out]
